vi "Get Item Resource.vi"(8 "error in (no error)":errorcluster, 10 "ItemName":string, 11 "Menu Data in":refnum<class "Menu Data.lvclass">) -> (0 "error out":errorcluster, 1 "Found?":bool, 2 "Resource":T2, 3 "Menu Data out":refnum<class "Menu Data.lvclass">, 5 "Languages":T1[](array[typedef]))   [LabVIEW 2013, in "SET Project Data.lvlib" / "Menu Data.lvclass"]
uses:
  Menu Data.lvclass
  Types/ProjFile_Resource Entry.ctl
  Types/ProjFile_Language Entry.ctl
  Menu Data.lvclass/Menu Data.ctl
  Resource Data Class/Resource Data.lvclass/Resource Data.ctl
  Resource Data Class/Read Languages.vi
  Resource Data Class/Resource Data.lvclass
  SET Project Data.lvlib
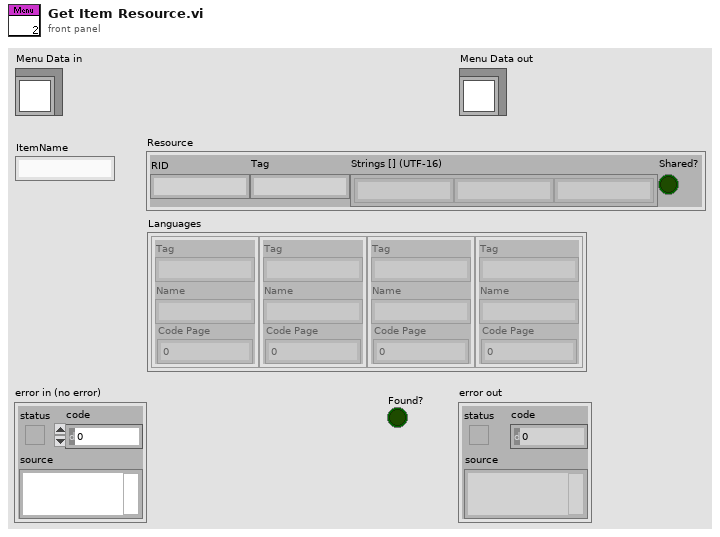
[diagram p1: front panel]
types:
  T1 = typedef "SET Project Data.lvlib/ProjFile_Language Entry.ctl" = cluster{"Tag":string, "Name":string, "Code Page":u16}
  T2 = typedef "SET Project Data.lvlib/ProjFile_Resource Entry.ctl" = cluster{"RID":string, "Tag":string, "Strings [] (UTF-16)":string[], "Shared?":bool}
  T3 = typedef "SET Project Data.lvlib/ProjFile_Language Data.ctl" = cluster{"Tag":string, "Name":string, "Code Page":u16}
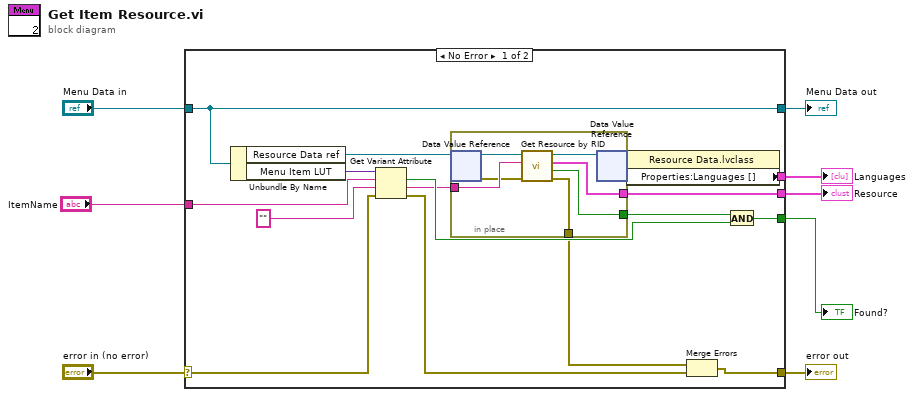
[diagram p0: block diagram]
diagram:
  n1 = case shown="No Error" "error in (no error)" {
    selector: "error in (no error)" -> [w20 w33]
    tunnel: [w9 w33] -> w7
    tunnel: [w24 w32] -> w5
    tunnel: "Menu Data in" -> [w24 w32]
    tunnel: "ItemName" -> [w22 _]
    tunnel: [w17 _] -> w3
    tunnel: [w16 _] -> w2
    tunnel: [w12 _] -> w1
    frame No Error {
      n2 = Unbundle By Name(w24) -> ("Resource Data ref"=w19:refnum<data-value>, "Menu Item LUT"=w23:variant)
      n3 = Get Variant Attribute(Variant=w23, name=w22, default value (empty Variant)="", error in=w20) -> (found=w14:bool, value=w13:string, error out=w10:errorcluster)  [unwired: 1 out]
      n4 = in-place {
        in-place-border: w13 -> [w29]
        in-place-border: [w28] -> w15
        in-place-border: [w25] -> w11
        in-place-border: [w27] -> w16
        n5 = in-place-dvr #1(w19) -> (w31:refnum<class "Resource Data.lvclass">, w26:errorcluster)
        n6 = call "Get Resource by RID.vi"("error in (no error)"=w26, "RID"=w29, "LangFile in"=w31) -> ("error out"=w25:errorcluster, "Found?"=w28:bool, "Resource"=w27:T2, "LangFile out"=w30:refnum<class "Resource Data.lvclass">)  [unwired: 4 in, 1 out]
        n7 = in-place-dvr #1(w30) -> (w18:refnum<data-value>)  [unwired: 1 out]
      }
      n8 = property class="Resource Data.lvclass"(reference=w18) -> ("Properties:Languages []"=w17:T3[])  [unwired: 1 in, 2 out]
      n9 = Merge Errors(w11, w10) -> (w9:errorcluster)
      n10 = And(x=w15, y=w14) -> (x .and. y?=w12:bool)
    }
    frame Error {
    }
  }
  "error out" <- w7
  "Menu Data out" <- w5
  "Found?" <- w1
  "Languages" <- w3
  "Resource" <- w2
